vi "檢測_Pattern_Sub.vi"(7 "Algorithm":i32(ring) items=["All", "Low Discrepancy Sampling", "Grayscale Value Pyramid", "Gradients Pyramid"], 8 "error in (no error)":errorcluster, 9 "ROI":T2, 10 "Image Dst":T1, 11 "Image Src":T1) -> (0 "error out":errorcluster, 3 "Template Image Out":T1)   [LabVIEW 2015]
uses:
  <vilib>/vision/Image Controls.llb/IMAQ Image.ctl
  <vilib>/vision/NI_Vision_Development_Module.lvlib
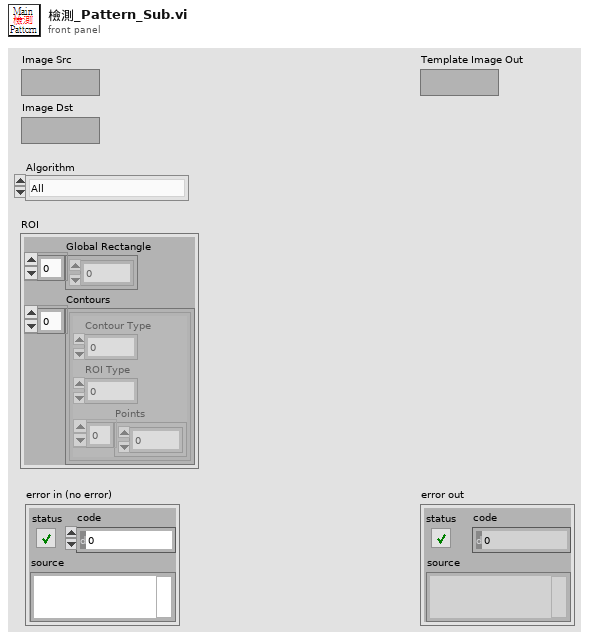
[diagram p1: front panel]
types:
  T1 = typedef "IMAQ Image.ctl" = refnum<image>
  T2 = cluster{"Global Rectangle":i32[], "Contours":cluster{"Contour Type":u32, "ROI Type":u32, "Points":i32[]}[]}
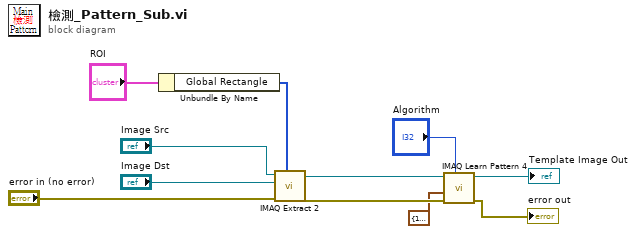
[diagram p0: block diagram]
diagram:
  n1 = Unbundle By Name("ROI") -> ("Global Rectangle"=w6:i32[])
  n2 = call "IMAQ Extract 2"("Optional Rectangle"=w6, "error in (no error)"="error in (no error)", "Image Dst"="Image Dst", "Image Src"="Image Src") -> ("error out"=w8:errorcluster, "Image Dst Out"=w9:T1)  [unwired: 6 in]
  n3 = call "IMAQ Learn Pattern 4"("Algorithm"="Algorithm", "error in (no error)"=w8, "Angle Range"=cluster{"Start Angle":sgl, "End Angle":sgl} {"Start Angle"=180.0, "End Angle"=-180.0}, "Image"=w9) -> ("error out"=→"error out":errorcluster, "Template Image Out"=→"Template Image Out":T1)  [unwired: 5 in, 1 out]
